vi "AIT 1553 - Create BM Message Name.vi"(0 "BM_Message":T1, 11 "error in (no error)":errorcluster) -> (4 "Message Name":string="CB_R_A_1E_Gun Control", 15 "error out":errorcluster)   [LabVIEW 2013]
uses:
  Controls/1553_BM_Message.ctl
  Controls/664 -Param.ctl
  AIT 664 Custom Device.lvlib
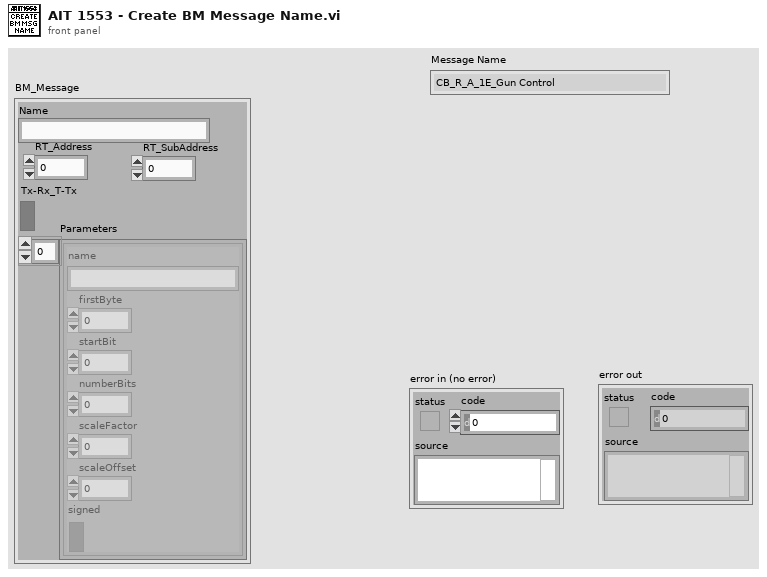
[diagram p1: front panel]
types:
  T1 = typedef "AIT 664 Custom Device.lvlib/1553_BM_Message.ctl" = cluster{"RT_Address":u8, "RT_SubAddress":u8, "Tx-Rx_T-Tx":bool, "Parameters":T2[], "Name":string}
  T2 = typedef "AIT 664 Custom Device.lvlib/664 -Param.ctl" = cluster{"name":string, "firstByte":i32, "startBit":i32, "numberBits":i32, "scaleFactor":dbl, "scaleOffset":dbl, "signed":bool}
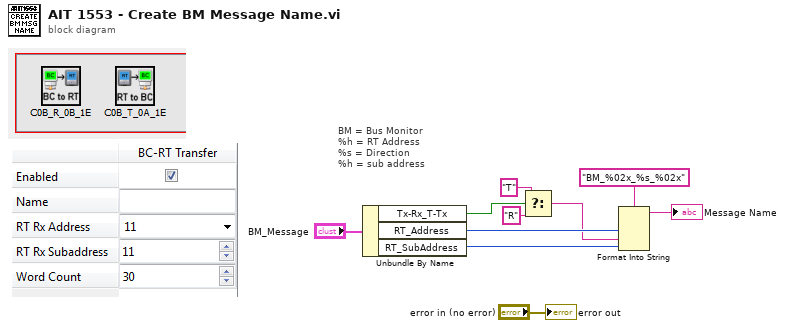
[diagram p0: block diagram]
diagram:
  # "BM = Bus Monitor\n%h = RT Address\n%s = Direction\n%h = sub address"
  n1 = Unbundle By Name("BM_Message") -> ("Tx-Rx_T-Tx"=w7:bool, "RT_Address"=w8:u8, "RT_SubAddress"=w3:u8)
  n2 = Select(t="T", s=w7, f="R") -> (s? t:f=w4:string)
  n3 = Format Into String(format string="BM_%02x_%s_%02x", w8, w4, w3) -> (resulting string=→"Message Name":string)  [unwired: 2 in, 1 out]
  "error out" <- "error in (no error)"
